vi "Dezimal-Matrix.vi"(1 "Color Box":u32(colorbox), 2 "string":string, 3 "number":dbl) -> (0 "output array":u32[][][](array[numeric]))   [LabVIEW 2021]
uses:
  ZahlenEnum.ctl
  <vilib>/Analysis/Matrix/Datatypes/RealMatrix.ctl
  <vilib>/Analysis/Matrix/NI_Matrix.lvlib
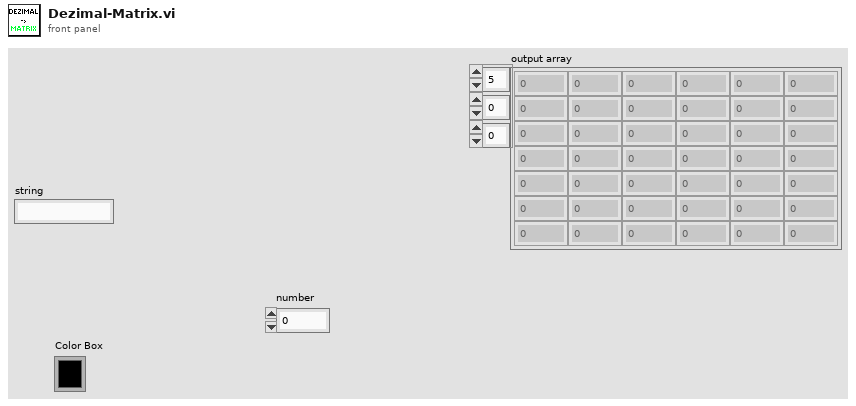
[diagram p1: front panel]
types:
  T1 = typedef "ZahlenEnum.ctl" = enum16{" ", ":", "%", "C", "°", ".", "9", "8", "7", "6", "5", "4", "3", "2", "1", "0"}
  T2 = typedef "NI_Matrix.lvlib/RealMatrix.ctl" = dbl[][]
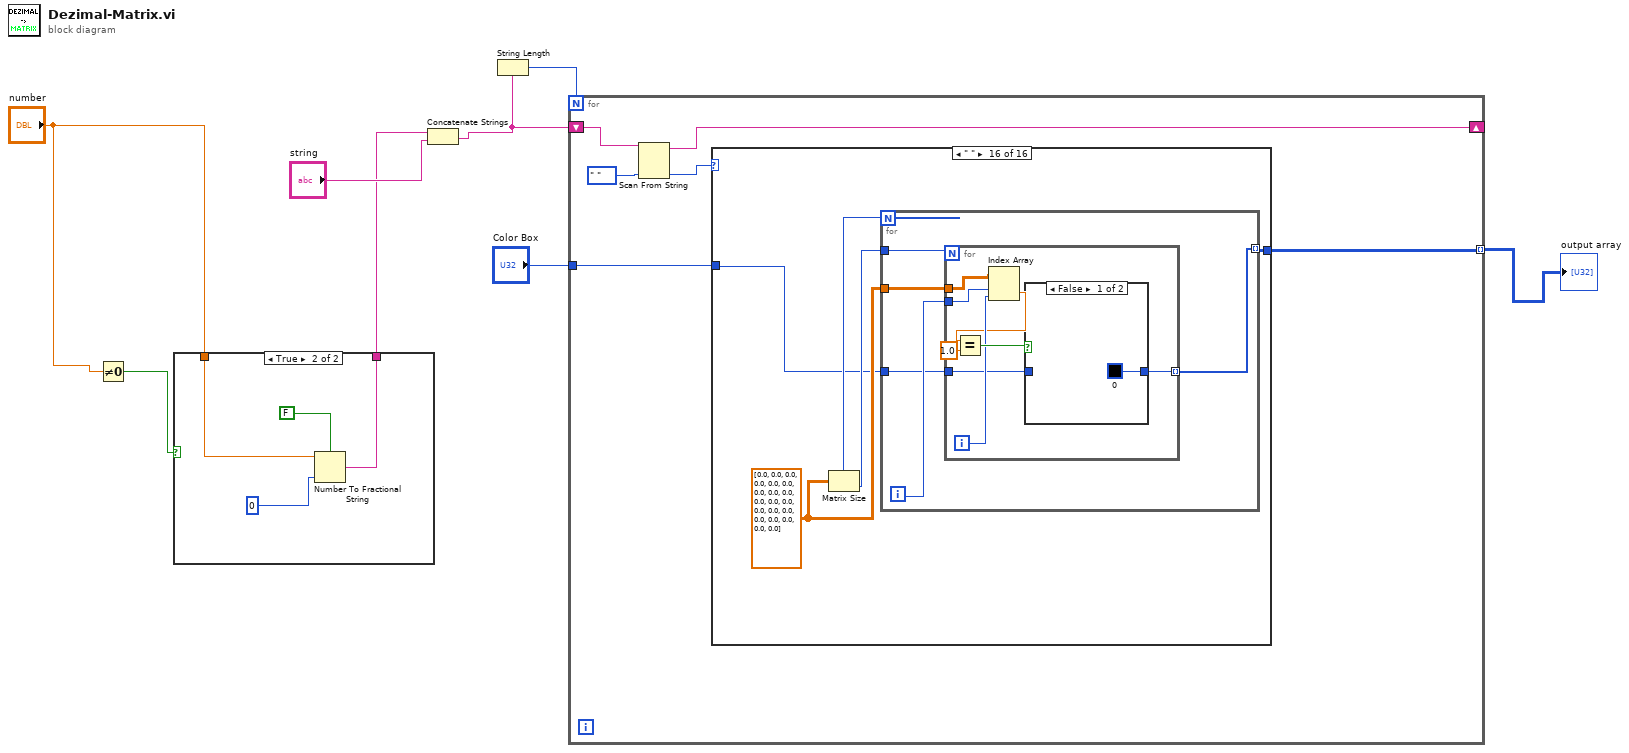
[diagram p0: block diagram]
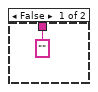
[diagram p2: hidden frame]
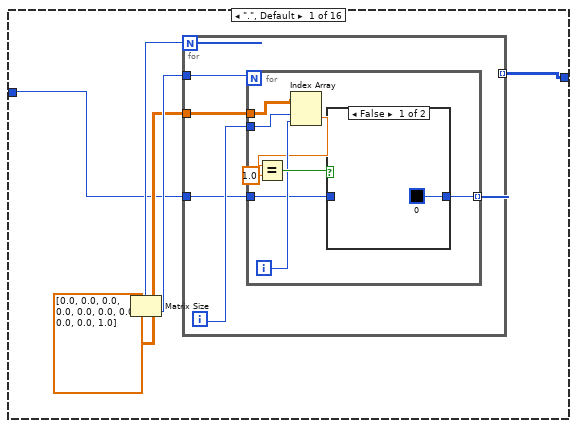
[diagram p3: hidden frame]
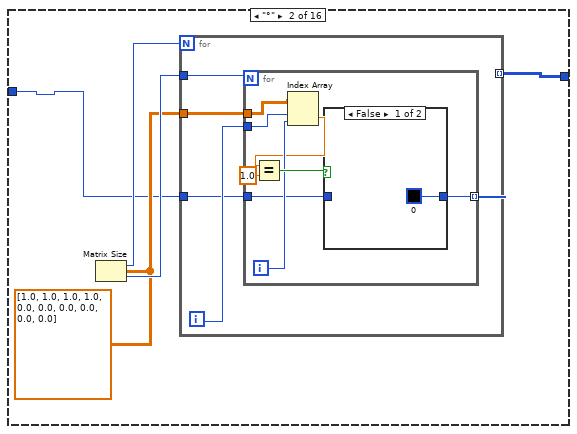
[diagram p5: hidden frame]
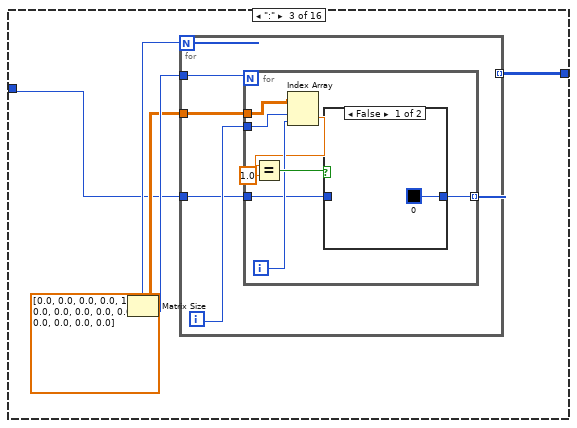
[diagram p7: hidden frame]
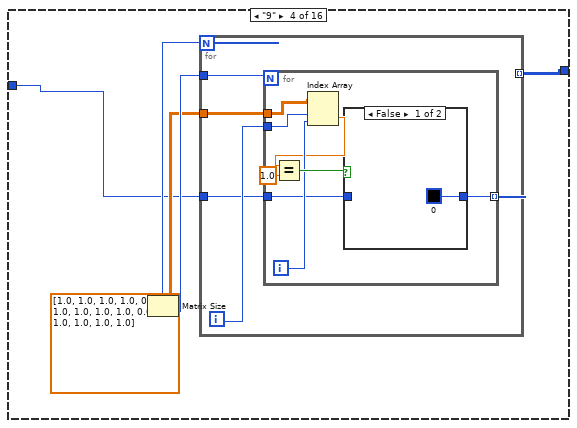
[diagram p9: hidden frame]
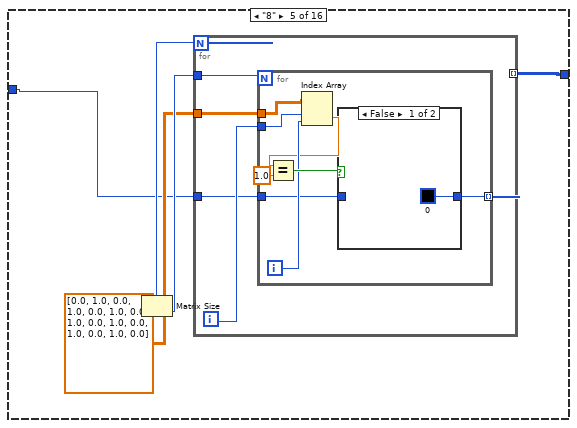
[diagram p11: hidden frame]
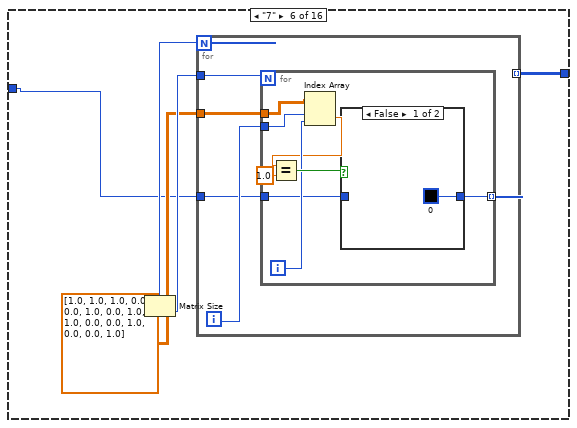
[diagram p13: hidden frame]
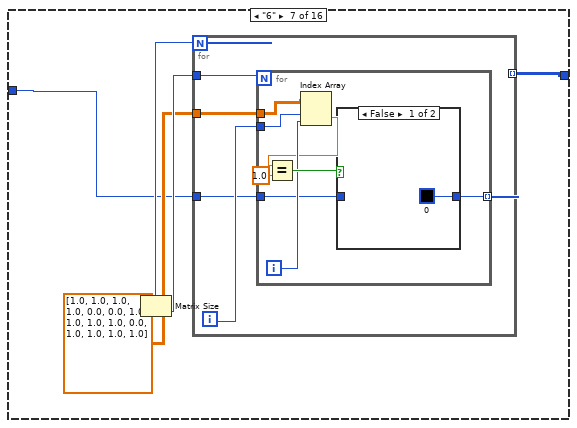
[diagram p15: hidden frame]
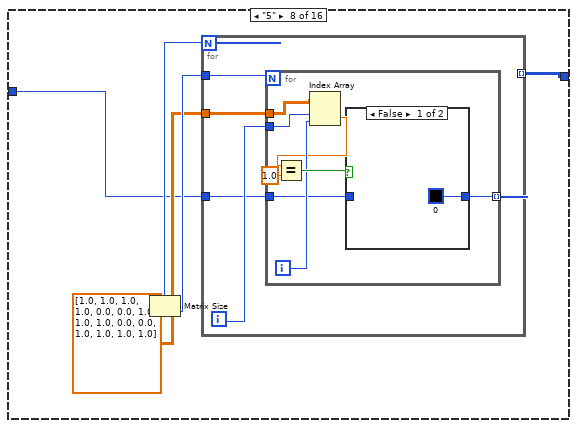
[diagram p17: hidden frame]
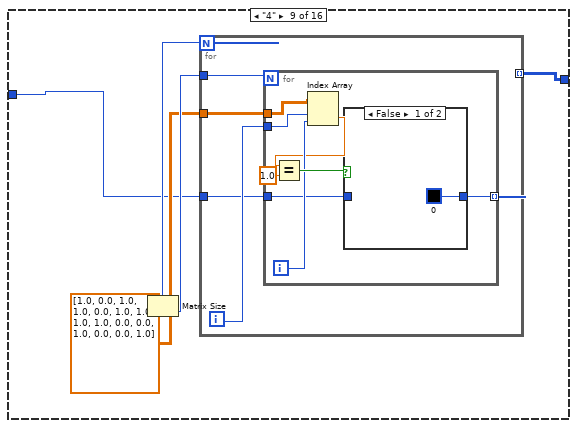
[diagram p19: hidden frame]
diagram:
  n1 = Not Equal To 0?(x="number") -> (x != 0?=w2:bool)
  n2 = case shown="True" w2 {
    tunnel: "number" -> [_ w11]
    tunnel: ["" w10] -> w3
    frame False {
    }
    frame True {
      n3 = Number To Fractional String(use system decimal point (T)=FALSE, number=w11, precision (6)=i16 0) -> (F-format string=w10:string)  [unwired: 1 in]
    }
  }
  n4 = Concatenate Strings(w3, "string") -> (w6:string)
  n5 = String Length(string=w6) -> (length=w4:i32)
  n6 = for {
    N: w4 -> [_]
    tunnel: "Color Box" -> [w17]
    tunnel: [w16] -> w7 mode=indexing
    shift-right: [w14] -> _
    shift-left: w6 -> [w15]
    n7 = Scan From String(input string=w15, default 1=ZahlenEnum." " ("Enum")) -> (remaining string=w14:string, output 1=w18:T1)  [unwired: 3 in, 2 out]
    n8 = case shown="\" \"" w18 {
      tunnel: w17 -> [w20 w41 w61 w81 w101 w121 w141 w161 w181 w201 w221 w241 w262 w281 w301 w321]
      tunnel: [w21 w40 w60 w80 w100 w120 w140 w160 w180 w200 w220 w240 w261 w280 w300 w320] -> w16
      frame ".", Default {
        w22 = T2 [[0.0, 0.0], [0.0, 0.0], [0.0, 0.0], [0.0, 0.0], [0.0, 1.0]] ("Real Matrix")
        n9 = Matrix Size(0:w22) -> (1:w24:i32, 2:w23:i32)
        n10 = for {
          N: w24 -> [_]
          tunnel: w23 -> [w29]
          tunnel: w22 -> [w27]
          tunnel: w20 -> [w26]
          tunnel: [w25] -> w21 mode=indexing
          i -> [w28]
          n11 = for {
            N: w29 -> [_]
            tunnel: w28 -> [w35]
            tunnel: w27 -> [w36]
            tunnel: w26 -> [w31]
            tunnel: [w30] -> w25 mode=indexing
            i -> [w34]
            n12 = Index Array(array=w36, index (row)=w35, index (col)=w34) -> (element=w33:dbl)
            n13 = Equal?(x=w33, y=1.0) -> (x = y?=w37:bool)
            n14 = case shown="False" w37 {
              tunnel: w31 -> [_ w39]
              tunnel: [u32 0 ("Color Box") w39] -> w30
              frame False {
              }
              frame True {
              }
            }
          }
        }
      }
      frame "°" {
        w42 = T2 [[1.0, 1.0], [1.0, 1.0], [0.0, 0.0], [0.0, 0.0], [0.0, 0.0]] ("Real Matrix")
        n15 = Matrix Size(0:w42) -> (1:w44:i32, 2:w43:i32)
        n16 = for {
          N: w44 -> [_]
          tunnel: w43 -> [w49]
          tunnel: w42 -> [w47]
          tunnel: w41 -> [w46]
          tunnel: [w45] -> w40 mode=indexing
          i -> [w48]
          n17 = for {
            N: w49 -> [_]
            tunnel: w48 -> [w55]
            tunnel: w47 -> [w56]
            tunnel: w46 -> [w51]
            tunnel: [w50] -> w45 mode=indexing
            i -> [w54]
            n18 = Index Array(array=w56, index (row)=w55, index (col)=w54) -> (element=w53:dbl)
            n19 = Equal?(x=w53, y=1.0) -> (x = y?=w57:bool)
            n20 = case shown="False" w57 {
              tunnel: w51 -> [_ w59]
              tunnel: [u32 0 ("Color Box") w59] -> w50
              frame False {
              }
              frame True {
              }
            }
          }
        }
      }
      frame ":" {
        w62 = T2 [[0.0, 0.0, 0.0], [0.0, 1.0, 0.0], [0.0, 0.0, 0.0], [0.0, 1.0, 0.0], [0.0, 0.0, 0.0]] ("Real Matrix")
        n21 = Matrix Size(0:w62) -> (1:w64:i32, 2:w63:i32)
        n22 = for {
          N: w64 -> [_]
          tunnel: w63 -> [w69]
          tunnel: w62 -> [w67]
          tunnel: w61 -> [w66]
          tunnel: [w65] -> w60 mode=indexing
          i -> [w68]
          n23 = for {
            N: w69 -> [_]
            tunnel: w68 -> [w75]
            tunnel: w67 -> [w76]
            tunnel: w66 -> [w71]
            tunnel: [w70] -> w65 mode=indexing
            i -> [w74]
            n24 = Index Array(array=w76, index (row)=w75, index (col)=w74) -> (element=w73:dbl)
            n25 = Equal?(x=w73, y=1.0) -> (x = y?=w77:bool)
            n26 = case shown="False" w77 {
              tunnel: w71 -> [_ w79]
              tunnel: [u32 0 ("Color Box") w79] -> w70
              frame False {
              }
              frame True {
              }
            }
          }
        }
      }
      frame "9" {
        w82 = T2 [[1.0, 1.0, 1.0], [1.0, 0.0, 1.0], [1.0, 1.0, 1.0], [0.0, 0.0, 1.0], [1.0, 1.0, 1.0]] ("Real Matrix")
        n27 = Matrix Size(0:w82) -> (1:w84:i32, 2:w83:i32)
        n28 = for {
          N: w84 -> [_]
          tunnel: w83 -> [w89]
          tunnel: w82 -> [w87]
          tunnel: w81 -> [w86]
          tunnel: [w85] -> w80 mode=indexing
          i -> [w88]
          n29 = for {
            N: w89 -> [_]
            tunnel: w88 -> [w95]
            tunnel: w87 -> [w96]
            tunnel: w86 -> [w91]
            tunnel: [w90] -> w85 mode=indexing
            i -> [w94]
            n30 = Index Array(array=w96, index (row)=w95, index (col)=w94) -> (element=w93:dbl)
            n31 = Equal?(x=w93, y=1.0) -> (x = y?=w97:bool)
            n32 = case shown="False" w97 {
              tunnel: w91 -> [_ w99]
              tunnel: [u32 0 ("Color Box") w99] -> w90
              frame False {
              }
              frame True {
              }
            }
          }
        }
      }
      frame "8" {
        w102 = T2 [[0.0, 1.0, 0.0], [1.0, 0.0, 1.0], [0.0, 1.0, 0.0], [1.0, 0.0, 1.0], [0.0, 1.0, 0.0]] ("Real Matrix")
        n33 = Matrix Size(0:w102) -> (1:w104:i32, 2:w103:i32)
        n34 = for {
          N: w104 -> [_]
          tunnel: w103 -> [w109]
          tunnel: w102 -> [w107]
          tunnel: w101 -> [w106]
          tunnel: [w105] -> w100 mode=indexing
          i -> [w108]
          n35 = for {
            N: w109 -> [_]
            tunnel: w108 -> [w115]
            tunnel: w107 -> [w116]
            tunnel: w106 -> [w111]
            tunnel: [w110] -> w105 mode=indexing
            i -> [w114]
            n36 = Index Array(array=w116, index (row)=w115, index (col)=w114) -> (element=w113:dbl)
            n37 = Equal?(x=w113, y=1.0) -> (x = y?=w117:bool)
            n38 = case shown="False" w117 {
              tunnel: w111 -> [_ w119]
              tunnel: [u32 0 ("Color Box") w119] -> w110
              frame False {
              }
              frame True {
              }
            }
          }
        }
      }
      frame "7" {
        w122 = T2 [[1.0, 1.0, 1.0], [0.0, 0.0, 1.0], [0.0, 1.0, 1.0], [0.0, 0.0, 1.0], [0.0, 0.0, 1.0]] ("Real Matrix")
        n39 = Matrix Size(0:w122) -> (1:w124:i32, 2:w123:i32)
        n40 = for {
          N: w124 -> [_]
          tunnel: w123 -> [w129]
          tunnel: w122 -> [w127]
          tunnel: w121 -> [w126]
          tunnel: [w125] -> w120 mode=indexing
          i -> [w128]
          n41 = for {
            N: w129 -> [_]
            tunnel: w128 -> [w135]
            tunnel: w127 -> [w136]
            tunnel: w126 -> [w131]
            tunnel: [w130] -> w125 mode=indexing
            i -> [w134]
            n42 = Index Array(array=w136, index (row)=w135, index (col)=w134) -> (element=w133:dbl)
            n43 = Equal?(x=w133, y=1.0) -> (x = y?=w137:bool)
            n44 = case shown="False" w137 {
              tunnel: w131 -> [_ w139]
              tunnel: [u32 0 ("Color Box") w139] -> w130
              frame False {
              }
              frame True {
              }
            }
          }
        }
      }
      frame "6" {
        w142 = T2 [[1.0, 1.0, 1.0], [1.0, 0.0, 0.0], [1.0, 1.0, 1.0], [1.0, 0.0, 1.0], [1.0, 1.0, 1.0]] ("Real Matrix")
        n45 = Matrix Size(0:w142) -> (1:w144:i32, 2:w143:i32)
        n46 = for {
          N: w144 -> [_]
          tunnel: w143 -> [w149]
          tunnel: w142 -> [w147]
          tunnel: w141 -> [w146]
          tunnel: [w145] -> w140 mode=indexing
          i -> [w148]
          n47 = for {
            N: w149 -> [_]
            tunnel: w148 -> [w155]
            tunnel: w147 -> [w156]
            tunnel: w146 -> [w151]
            tunnel: [w150] -> w145 mode=indexing
            i -> [w154]
            n48 = Index Array(array=w156, index (row)=w155, index (col)=w154) -> (element=w153:dbl)
            n49 = Equal?(x=w153, y=1.0) -> (x = y?=w157:bool)
            n50 = case shown="False" w157 {
              tunnel: w151 -> [_ w159]
              tunnel: [u32 0 ("Color Box") w159] -> w150
              frame False {
              }
              frame True {
              }
            }
          }
        }
      }
      frame "5" {
        w162 = T2 [[1.0, 1.0, 1.0], [1.0, 0.0, 0.0], [1.0, 1.0, 1.0], [0.0, 0.0, 1.0], [1.0, 1.0, 1.0]] ("Real Matrix")
        n51 = Matrix Size(0:w162) -> (1:w164:i32, 2:w163:i32)
        n52 = for {
          N: w164 -> [_]
          tunnel: w163 -> [w169]
          tunnel: w162 -> [w167]
          tunnel: w161 -> [w166]
          tunnel: [w165] -> w160 mode=indexing
          i -> [w168]
          n53 = for {
            N: w169 -> [_]
            tunnel: w168 -> [w175]
            tunnel: w167 -> [w176]
            tunnel: w166 -> [w171]
            tunnel: [w170] -> w165 mode=indexing
            i -> [w174]
            n54 = Index Array(array=w176, index (row)=w175, index (col)=w174) -> (element=w173:dbl)
            n55 = Equal?(x=w173, y=1.0) -> (x = y?=w177:bool)
            n56 = case shown="False" w177 {
              tunnel: w171 -> [_ w179]
              tunnel: [u32 0 ("Color Box") w179] -> w170
              frame False {
              }
              frame True {
              }
            }
          }
        }
      }
      frame "4" {
        w182 = T2 [[1.0, 0.0, 1.0], [1.0, 0.0, 1.0], [1.0, 1.0, 1.0], [0.0, 0.0, 1.0], [0.0, 0.0, 1.0]] ("Real Matrix")
        n57 = Matrix Size(0:w182) -> (1:w184:i32, 2:w183:i32)
        n58 = for {
          N: w184 -> [_]
          tunnel: w183 -> [w189]
          tunnel: w182 -> [w187]
          tunnel: w181 -> [w186]
          tunnel: [w185] -> w180 mode=indexing
          i -> [w188]
          n59 = for {
            N: w189 -> [_]
            tunnel: w188 -> [w195]
            tunnel: w187 -> [w196]
            tunnel: w186 -> [w191]
            tunnel: [w190] -> w185 mode=indexing
            i -> [w194]
            n60 = Index Array(array=w196, index (row)=w195, index (col)=w194) -> (element=w193:dbl)
            n61 = Equal?(x=w193, y=1.0) -> (x = y?=w197:bool)
            n62 = case shown="False" w197 {
              tunnel: w191 -> [_ w199]
              tunnel: [u32 0 ("Color Box") w199] -> w190
              frame False {
              }
              frame True {
              }
            }
          }
        }
      }
      frame "3" {
        w202 = T2 [[1.0, 1.0, 1.0], [0.0, 0.0, 1.0], [1.0, 1.0, 1.0], [0.0, 0.0, 1.0], [1.0, 1.0, 1.0]] ("Real Matrix")
        n63 = Matrix Size(0:w202) -> (1:w204:i32, 2:w203:i32)
        n64 = for {
          N: w204 -> [_]
          tunnel: w203 -> [w209]
          tunnel: w202 -> [w207]
          tunnel: w201 -> [w206]
          tunnel: [w205] -> w200 mode=indexing
          i -> [w208]
          n65 = for {
            N: w209 -> [_]
            tunnel: w208 -> [w215]
            tunnel: w207 -> [w216]
            tunnel: w206 -> [w211]
            tunnel: [w210] -> w205 mode=indexing
            i -> [w214]
            n66 = Index Array(array=w216, index (row)=w215, index (col)=w214) -> (element=w213:dbl)
            n67 = Equal?(x=w213, y=1.0) -> (x = y?=w217:bool)
            n68 = case shown="False" w217 {
              tunnel: w211 -> [_ w219]
              tunnel: [u32 0 ("Color Box") w219] -> w210
              frame False {
              }
              frame True {
              }
            }
          }
        }
      }
      frame "2" {
        w222 = T2 [[1.0, 1.0, 0.0], [0.0, 0.0, 1.0], [1.0, 1.0, 1.0], [1.0, 0.0, 0.0], [0.0, 1.0, 1.0]] ("Real Matrix")
        n69 = Matrix Size(0:w222) -> (1:w224:i32, 2:w223:i32)
        n70 = for {
          N: w224 -> [_]
          tunnel: w223 -> [w229]
          tunnel: w222 -> [w227]
          tunnel: w221 -> [w226]
          tunnel: [w225] -> w220 mode=indexing
          i -> [w228]
          n71 = for {
            N: w229 -> [_]
            tunnel: w228 -> [w235]
            tunnel: w227 -> [w236]
            tunnel: w226 -> [w231]
            tunnel: [w230] -> w225 mode=indexing
            i -> [w234]
            n72 = Index Array(array=w236, index (row)=w235, index (col)=w234) -> (element=w233:dbl)
            n73 = Equal?(x=w233, y=1.0) -> (x = y?=w237:bool)
            n74 = case shown="False" w237 {
              tunnel: w231 -> [_ w239]
              tunnel: [u32 0 ("Color Box") w239] -> w230
              frame False {
              }
              frame True {
              }
            }
          }
        }
      }
      frame "1" {
        w242 = T2 [[0.0, 1.0, 1.0], [0.0, 0.0, 1.0], [0.0, 0.0, 1.0], [0.0, 0.0, 1.0], [0.0, 0.0, 1.0]] ("Real Matrix")
        n75 = Matrix Size(0:w242) -> (1:w244:i32, 2:w243:i32)
        n76 = for {
          N: w244 -> [_]
          tunnel: w243 -> [w249]
          tunnel: w242 -> [w247]
          tunnel: w241 -> [w246]
          tunnel: [w245] -> w240 mode=indexing
          i -> [w248]
          n77 = for {
            N: w249 -> [_]
            tunnel: w248 -> [w255]
            tunnel: w247 -> [w256]
            tunnel: w246 -> [w251]
            tunnel: [w250] -> w245 mode=indexing
            i -> [w254]
            n78 = Index Array(array=w256, index (row)=w255, index (col)=w254) -> (element=w253:dbl)
            n79 = Equal?(x=w253, y=1.0) -> (x = y?=w257:bool)
            n80 = case shown="False" w257 {
              tunnel: w251 -> [_ w259]
              tunnel: [u32 0 ("Color Box") w259] -> w250
              frame False {
              }
              frame True {
              }
            }
          }
        }
      }
      frame "0" {
        w260 = T2 [[0.0, 1.0, 0.0], [1.0, 0.0, 1.0], [1.0, 0.0, 1.0], [1.0, 0.0, 1.0], [0.0, 1.0, 0.0]] ("Real Matrix")
        n81 = Matrix Size(0:w260) -> (1:w264:i32, 2:w263:i32)
        n82 = for {
          N: w264 -> [_]
          tunnel: w263 -> [w269]
          tunnel: w260 -> [w267]
          tunnel: w262 -> [w266]
          tunnel: [w265] -> w261 mode=indexing
          i -> [w268]
          n83 = for {
            N: w269 -> [_]
            tunnel: w268 -> [w275]
            tunnel: w267 -> [w276]
            tunnel: w266 -> [w271]
            tunnel: [w270] -> w265 mode=indexing
            i -> [w274]
            n84 = Index Array(array=w276, index (row)=w275, index (col)=w274) -> (element=w273:dbl)
            n85 = Equal?(x=w273, y=1.0) -> (x = y?=w277:bool)
            n86 = case shown="False" w277 {
              tunnel: w271 -> [_ w279]
              tunnel: [u32 0 ("Color Box") w279] -> w270
              frame False {
              }
              frame True {
              }
            }
          }
        }
      }
      frame "C" {
        w282 = T2 [[0.0, 1.0, 1.0], [1.0, 0.0, 0.0], [1.0, 0.0, 0.0], [1.0, 0.0, 0.0], [0.0, 1.0, 1.0]] ("Real Matrix")
        n87 = Matrix Size(0:w282) -> (1:w284:i32, 2:w283:i32)
        n88 = for {
          N: w284 -> [_]
          tunnel: w283 -> [w289]
          tunnel: w282 -> [w287]
          tunnel: w281 -> [w286]
          tunnel: [w285] -> w280 mode=indexing
          i -> [w288]
          n89 = for {
            N: w289 -> [_]
            tunnel: w288 -> [w295]
            tunnel: w287 -> [w296]
            tunnel: w286 -> [w291]
            tunnel: [w290] -> w285 mode=indexing
            i -> [w294]
            n90 = Index Array(array=w296, index (row)=w295, index (col)=w294) -> (element=w293:dbl)
            n91 = Equal?(x=w293, y=1.0) -> (x = y?=w297:bool)
            n92 = case shown="False" w297 {
              tunnel: w291 -> [_ w299]
              tunnel: [u32 0 ("Color Box") w299] -> w290
              frame False {
              }
              frame True {
              }
            }
          }
        }
      }
      frame "%" {
        w302 = T2 [[1.0, 0.0, 1.0], [0.0, 0.0, 1.0], [0.0, 1.0, 0.0], [1.0, 0.0, 0.0], [1.0, 0.0, 1.0]] ("Real Matrix")
        n93 = Matrix Size(0:w302) -> (1:w304:i32, 2:w303:i32)
        n94 = for {
          N: w304 -> [_]
          tunnel: w303 -> [w309]
          tunnel: w302 -> [w307]
          tunnel: w301 -> [w306]
          tunnel: [w305] -> w300 mode=indexing
          i -> [w308]
          n95 = for {
            N: w309 -> [_]
            tunnel: w308 -> [w315]
            tunnel: w307 -> [w316]
            tunnel: w306 -> [w311]
            tunnel: [w310] -> w305 mode=indexing
            i -> [w314]
            n96 = Index Array(array=w316, index (row)=w315, index (col)=w314) -> (element=w313:dbl)
            n97 = Equal?(x=w313, y=1.0) -> (x = y?=w317:bool)
            n98 = case shown="False" w317 {
              tunnel: w311 -> [_ w319]
              tunnel: [u32 0 ("Color Box") w319] -> w310
              frame False {
              }
              frame True {
              }
            }
          }
        }
      }
      frame " " {
        w322 = T2 [[0.0, 0.0, 0.0, 0.0], [0.0, 0.0, 0.0, 0.0], [0.0, 0.0, 0.0, 0.0], [0.0, 0.0, 0.0, 0.0], [0.0, 0.0, 0.0, 0.0]] ("Real Matrix")
        n99 = Matrix Size(0:w322) -> (1:w323:i32, 2:w324:i32)
        n100 = for {
          N: w323 -> [_]
          tunnel: w324 -> [w329]
          tunnel: w322 -> [w327]
          tunnel: w321 -> [w326]
          tunnel: [w325] -> w320 mode=indexing
          i -> [w328]
          n101 = for {
            N: w329 -> [_]
            tunnel: w328 -> [w335]
            tunnel: w327 -> [w336]
            tunnel: w326 -> [w331]
            tunnel: [w330] -> w325 mode=indexing
            i -> [w334]
            n102 = Index Array(array=w336, index (row)=w335, index (col)=w334) -> (element=w333:dbl)
            n103 = Equal?(x=w333, y=1.0) -> (x = y?=w337:bool)
            n104 = case shown="False" w337 {
              tunnel: w331 -> [_ w339]
              tunnel: [u32 0 ("Color Box") w339] -> w330
              frame False {
              }
              frame True {
              }
            }
          }
        }
      }
    }
  }
  "output array" <- w7
